vi "AMZ_S3_Create Headers v4.vi"(5 "request headers":cluster{"item":string, "value":string}[](array[cluster]), 7 "RequestBody Payload":string, 8 "date/time string":string, 9 "Host":string, 10 "Client Handle In":T1) -> (1 "Signed Headers":string, 2 "canonical headers":string, 3 "Client Handle Out":T1)   [LabVIEW 2015, in "LV Interface for Amazon S3.lvlib"]
uses:
  LV Interface for Amazon S3.lvlib
  <vilib>/httpClient/ClientHandle.ctl
  <vilib>/httpClient/LabVIEWHTTPClient.lvlib
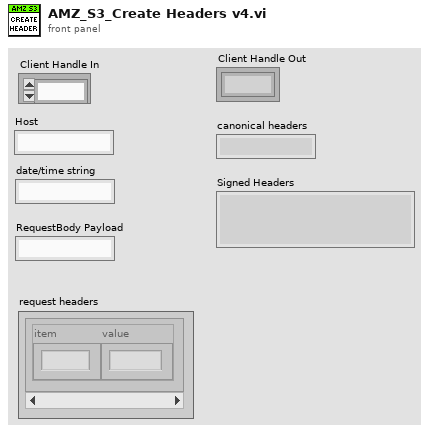
[diagram p1: front panel]
types:
  T1 = typedef "LabVIEWHTTPClient.lvlib/ClientHandle.ctl" = refnum<k1>
  T2 = cluster{"item":string, "RequestBody Payload":string}[]
  T3 = cluster{string, "item":string, "RequestBody Payload":string}
  T4 = cluster{string, "item":string, "RequestBody Payload":string}[]
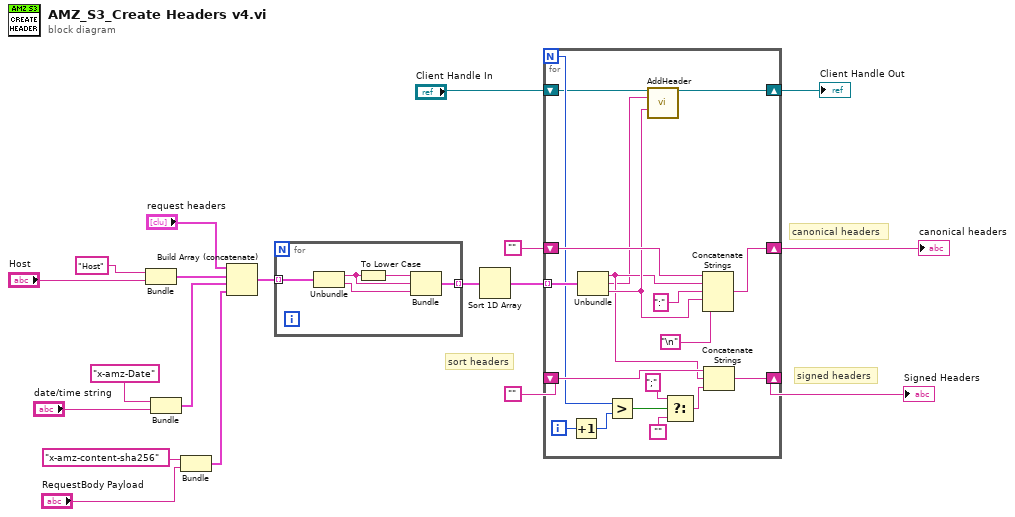
[diagram p0: block diagram]
diagram:
  # "signed headers"
  # "sort headers"
  # "canonical headers"
  n1 = Bundle("Host", "Host"="Host") -> (w11:cluster{string, "Host":string})  [unwired: 1 in]
  n2 = Bundle("x-amz-Date", "date/time string"="date/time string") -> (w13:cluster{string, "date/time string":string})  [unwired: 1 in]
  n3 = Bundle("x-amz-content-sha256", "RequestBody Payload"="RequestBody Payload") -> (w17:cluster{string, "RequestBody Payload":string})  [unwired: 1 in]
  n4 = Build Array (concatenate)("request headers", w11, w13, w17) -> (w3:T2)
  n5 = for {
    tunnel: w3 -> [w24] mode=indexing
    tunnel: [w21] -> w2 mode=indexing
    n6 = Unbundle(w24) -> ("item"=w22:string, "RequestBody Payload"=w20:string)
    n7 = To Lower Case(string=w22) -> (all lower case string=w23:string)
    n8 = Bundle(w23, "item"=w22, "RequestBody Payload"=w20) -> (w21:T3)  [unwired: 1 in]
  }
  n9 = Sort 1D Array(array=w2) -> (sorted array=w9:T4)
  n10 = for {
    N -> [w36]
    tunnel: w9 -> [w43] mode=indexing
    shift-right: [w39] -> w6
    shift-left: "" -> [w40]
    shift-right: [w38] -> w5
    shift-left: "" -> [w37]
    shift-right: [w30] -> w4
    shift-left: "Client Handle In" -> [w31]
    i -> [w29]
    n11 = Increment(x=w29) -> (x+1=w28:i32)
    n12 = Unbundle(w43) -> (w26:string, "item"=w25:string, "RequestBody Payload"=w27:string)
    n13 = Greater?(x=w36, y=w28) -> (0:w35:bool)
    n14 = call <vilib>:"AddHeader.vi"("client handle"=w31, "header"=w25, "value"=w27) -> ("client handle out"=w30:T1)  [unwired: 11 in, 1 out]
    n15 = Select(t=";", s=w35, f="") -> (s? t:f=w32:string)
    n16 = Concatenate Strings(w40, w26, ":", w27, "\n") -> (w39:string)
    n17 = Concatenate Strings(w37, w26, w32) -> (w38:string)
  }
  "canonical headers" <- w6
  "Signed Headers" <- w5
  "Client Handle Out" <- w4
